vi "Configure Sync Burst Sine.vi"(0 "VISA resource name":refnum<visa-resource-name>, 1 "High Amplitude Time (1 cyc)":dbl=1.0, 2 "Enable Waveform (T: Enable)":bool=TRUE, 3 "Enable EQ Output Modification (T: Enable)":bool=TRUE, 5 "Channel (0: A)":i32(ring) items=["A", "B"], 7 "Amplitude (0 Vrms)":dbl, 9 "Frequency (10 Hz)":dbl=10.0, 11 "error in (no error)":errorcluster, 12 "Low Amplitude (0 %)":dbl, 13 "Burst Period (2 cyc)":dbl=2.0, 14 "Trigger Mode (0: sbInternal)":i32(ring) items=["sbInternal", "sbExtTriggered", "sbExtGated"]) -> (4 "VISA resource name out":refnum<visa-resource-name>, 15 "error out":errorcluster)   [LabVIEW 2014, in "Stanford Research SR1.lvlib"]
doc: "Configures the attributes for the Analog Generator Sync Curst Sine."
uses:
  Stanford Research SR1.lvlib
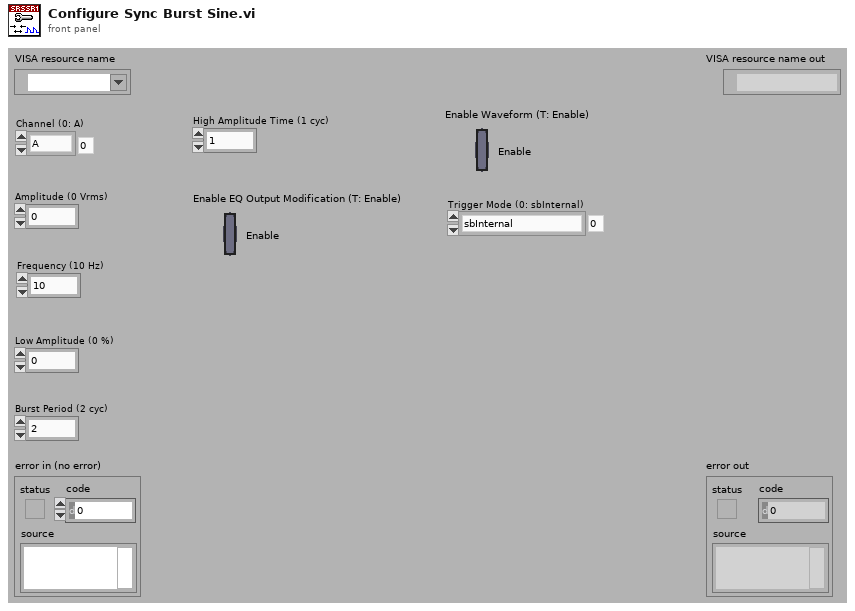
[diagram p1: front panel]
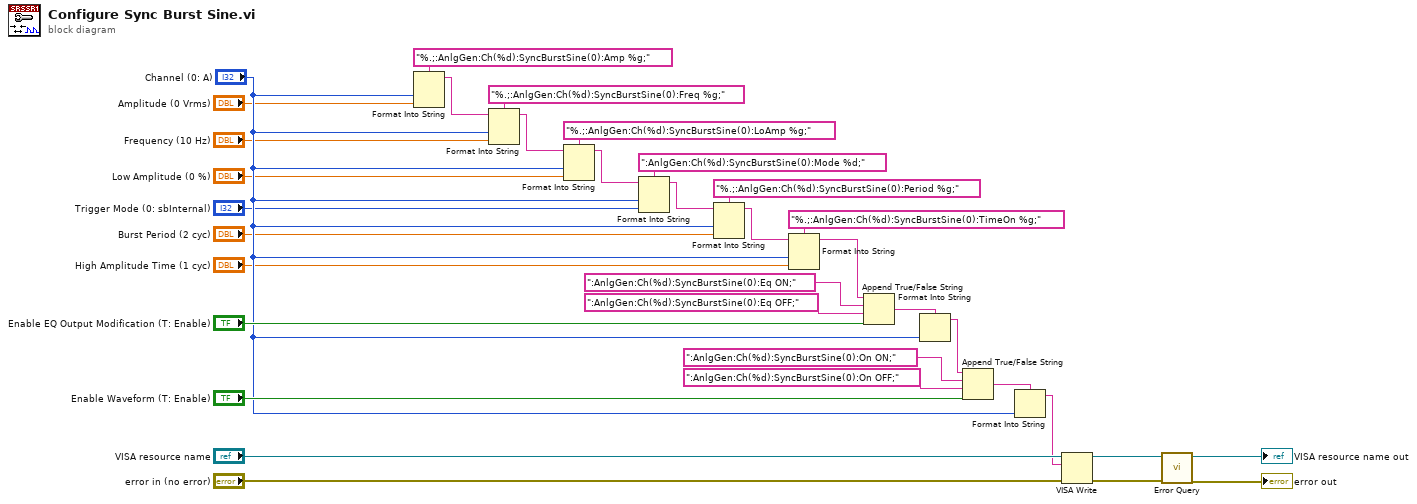
[diagram p0: block diagram]
diagram:
  n1 = Format Into String(format string="%.;:AnlgGen:Ch(%d):SyncBurstSine(0):Amp %g;", "Channel (0: A)", "Amplitude (0 Vrms)") -> (resulting string=w34:string)  [unwired: 2 in, 1 out]
  n2 = Format Into String(format string="%.;:AnlgGen:Ch(%d):SyncBurstSine(0):Freq %g;", initial string=w34, "Channel (0: A)", "Frequency (10 Hz)") -> (resulting string=w32:string)  [unwired: 1 in, 1 out]
  n3 = Format Into String(format string="%.;:AnlgGen:Ch(%d):SyncBurstSine(0):LoAmp %g;", initial string=w32, "Channel (0: A)", "Low Amplitude (0 %)") -> (resulting string=w30:string)  [unwired: 1 in, 1 out]
  n4 = Format Into String(format string=":AnlgGen:Ch(%d):SyncBurstSine(0):Mode %d;", initial string=w30, "Channel (0: A)", "Trigger Mode (0: sbInternal)") -> (resulting string=w28:string)  [unwired: 1 in, 1 out]
  n5 = Format Into String(format string="%.;:AnlgGen:Ch(%d):SyncBurstSine(0):Period %g;", initial string=w28, "Channel (0: A)", "Burst Period (2 cyc)") -> (resulting string=w26:string)  [unwired: 1 in, 1 out]
  n6 = Format Into String(format string="%.;:AnlgGen:Ch(%d):SyncBurstSine(0):TimeOn %g;", initial string=w26, "Channel (0: A)", "High Amplitude Time (1 cyc)") -> (resulting string=w24:string)  [unwired: 1 in, 1 out]
  n7 = Append True/False String(1:"Enable EQ Output Modification (T: Enable)", 2:":AnlgGen:Ch(%d):SyncBurstSine(0):Eq OFF;", 3:":AnlgGen:Ch(%d):SyncBurstSine(0):Eq ON;", 4:w24) -> (0:w11:string)
  n8 = Format Into String(format string=w11, "Channel (0: A)") -> (resulting string=w10:string)  [unwired: 2 in, 1 out]
  n9 = Append True/False String(1:"Enable Waveform (T: Enable)", 2:":AnlgGen:Ch(%d):SyncBurstSine(0):On OFF;", 3:":AnlgGen:Ch(%d):SyncBurstSine(0):On ON;", 4:w10) -> (0:w9:string)
  n10 = Format Into String(format string=w9, "Channel (0: A)") -> (resulting string=w8:string)  [unwired: 2 in, 1 out]
  n11 = VISA Write(VISA resource name="VISA resource name", write buffer=w8, error in (no error)="error in (no error)") -> (VISA resource name out=w15:refnum<visa-resource-name>, error out=w14:errorcluster)  [unwired: 1 out]
  n12 = call "Error Query.vi"("error in (no error)"=w14, "VISA resource name"=w15) -> ("error out"=→"error out":errorcluster, "VISA resource name out"=→"VISA resource name out":refnum<visa-resource-name>)  [unwired: 6 in, 2 out]
